vi "Download TBD file.vi"(8 "error in (no error)":errorcluster caption="错误输入（无错误）", 10 "TBC File Name":string="E100_TS2_23_90_V3.0.tbc", 11 "VISA资源名称":refnum<visa-resource-name>="COM1") -> (0 "错误输出":errorcluster, 2 "CMD In":string[](array[string]), 3 "Result":bool)   [LabVIEW 2013]
uses:
  C:/Program Files/National Instruments/LabVIEW 2013/examples/Instrument IO/Serial/support/Serial - Settings.ctl
  <vilib>/Instr/_visa.llb/VISA Configure Serial Port (Instr).vi
panel:
  out "读取缓冲区":string
  in  "文件路径（使用对话框）":path=path "E:/TBOX NEW/E100_TS2_23_90_V3.0.tbc"
  in  "TBC File Name 2":string="E100_TS2_23_90_V3.0.tbc"
  out "数组 2":bool[](array[boolean])
  out "添加的路径":path
  out "Feedback":string[](array[string])
  out "数组":string[](array[string])
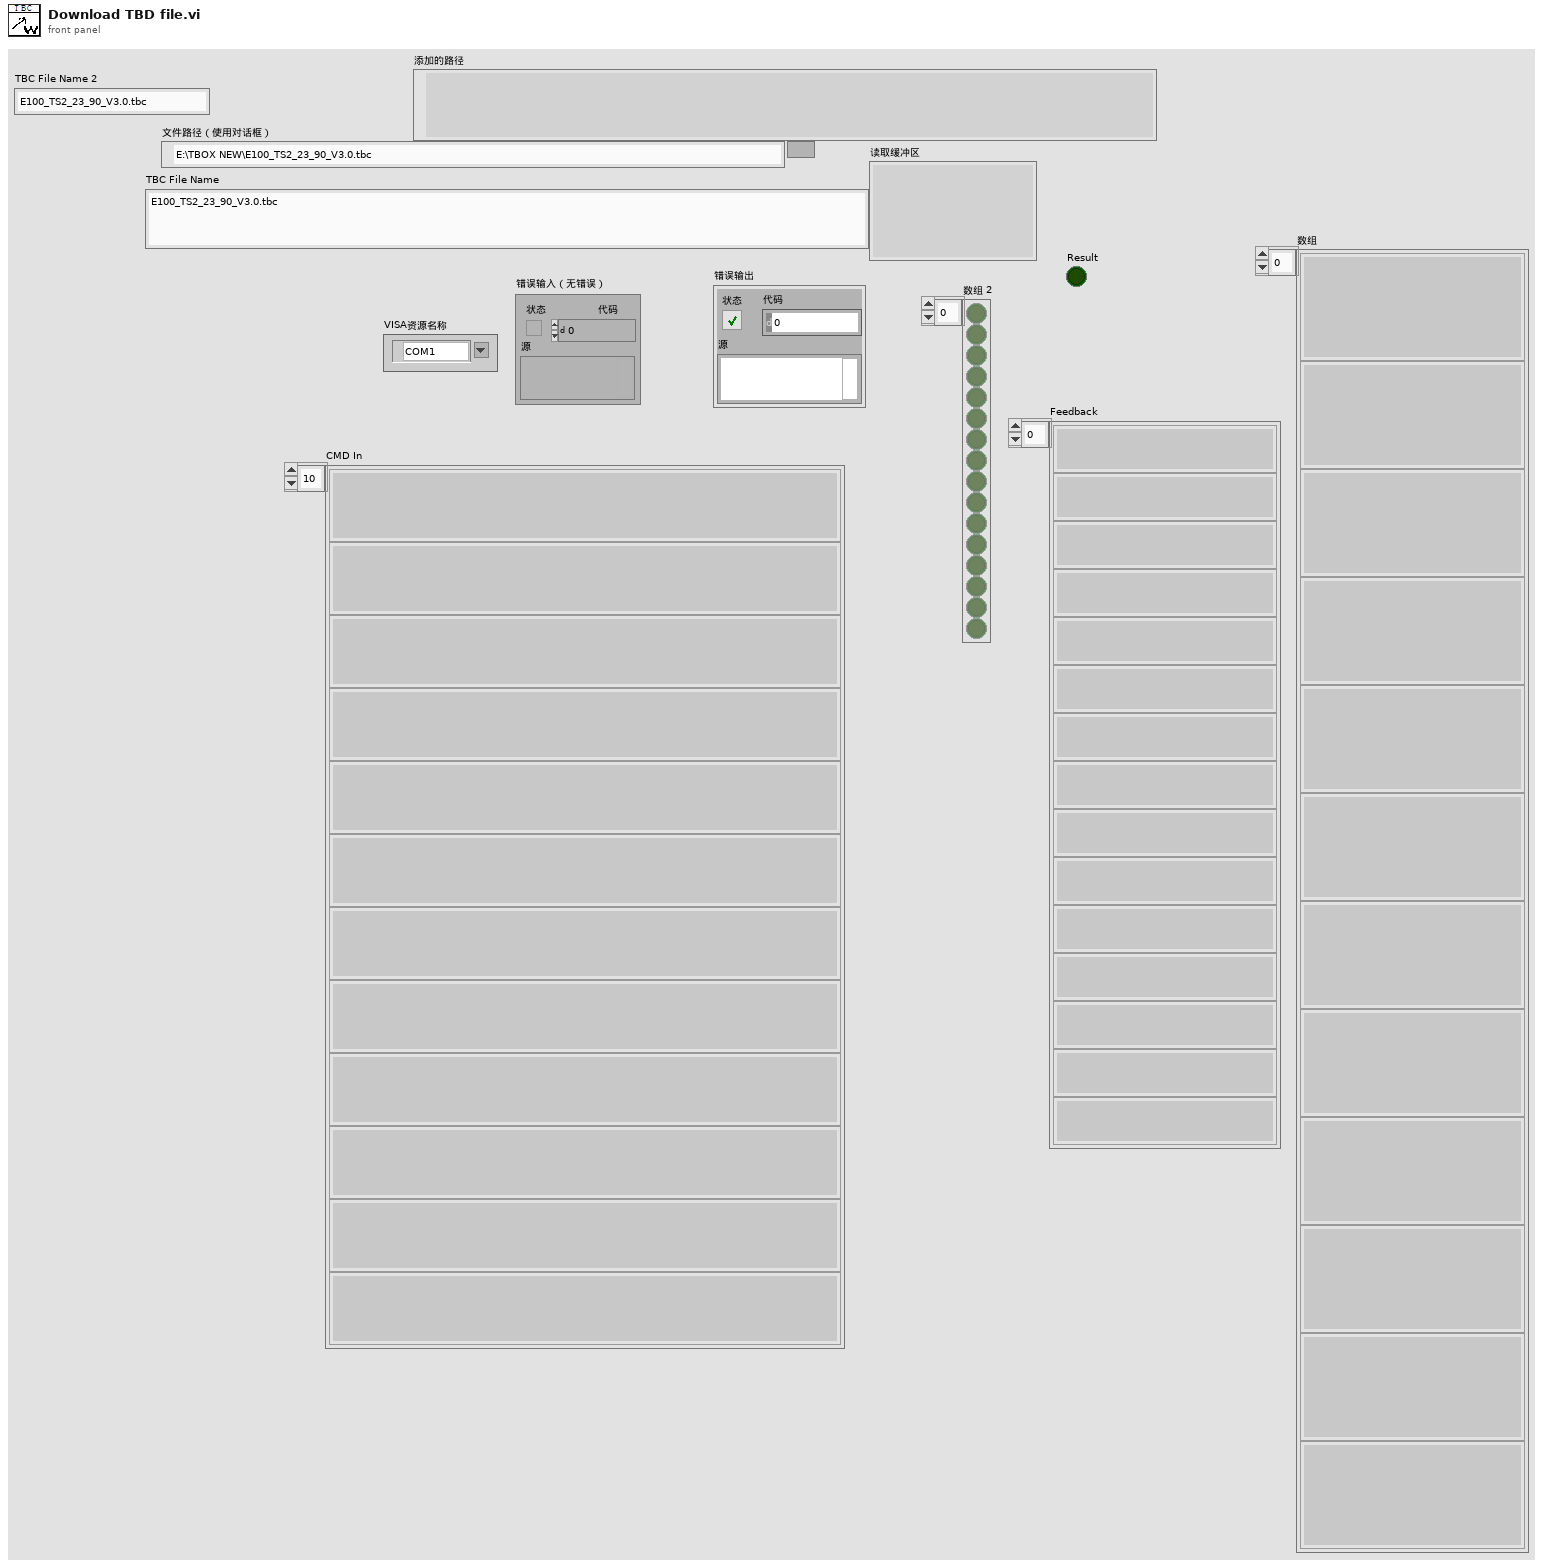
[diagram p1: front panel]
types:
  T1 = enum32{"invalid app kind", "Development System", "Run Time System", "Student Edition", "Embedded LabVIEW", "Evaluation", "Custom"}
  T2 = typedef "Serial - Settings.ctl" = cluster{"波特率":u32, "数据比特":u16, "奇偶":enum16{"None", "Odd", "Even", "Mark", "Space"}, "停止位":u16, "流控制":u16}
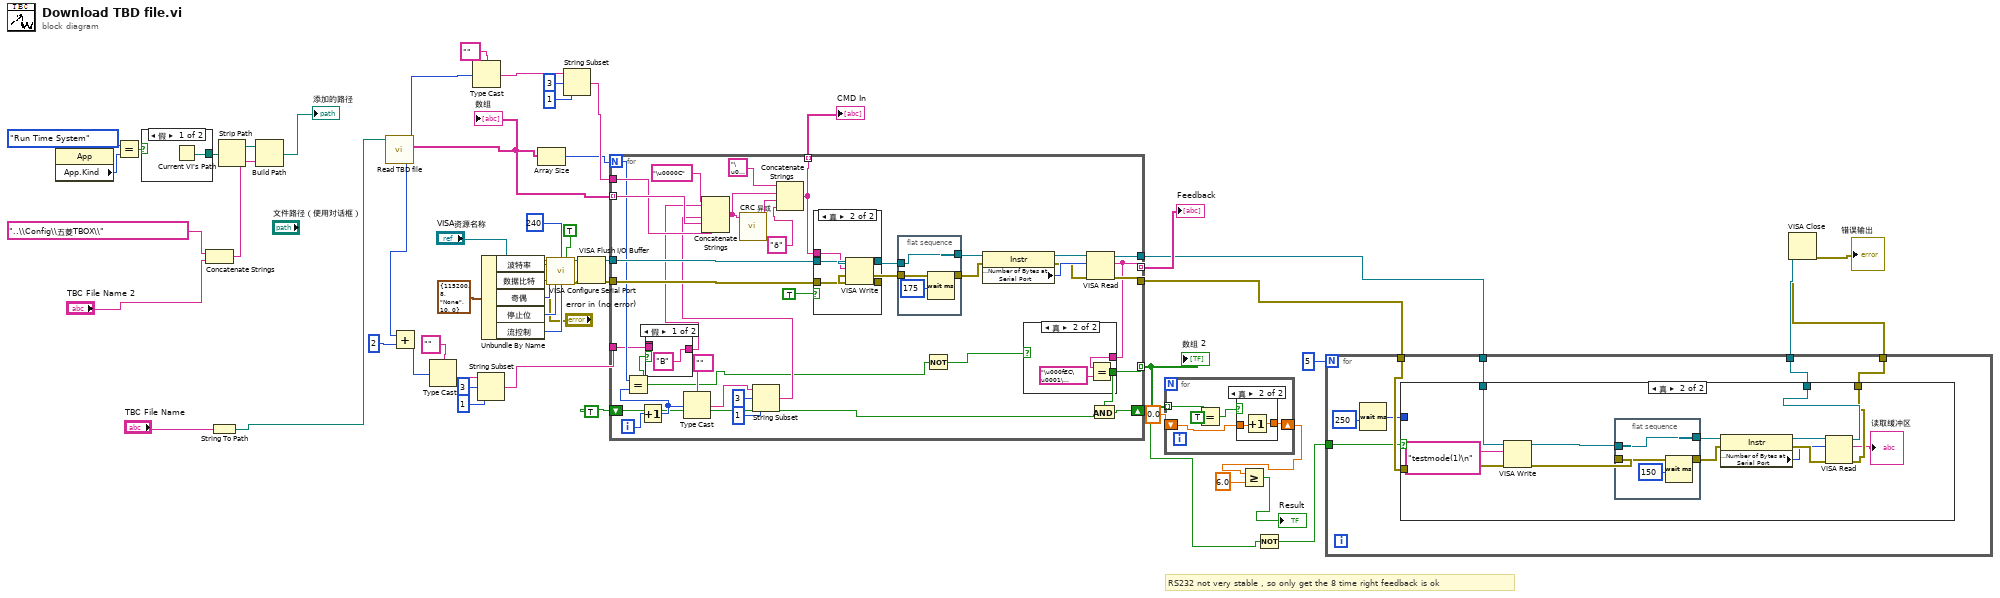
[diagram p0: block diagram]
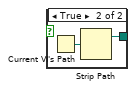
[diagram p4: hidden frame]
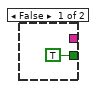
[diagram p5: hidden frame]
diagram:
  # "RS232 not very stable , so only get the 8 time right feedback is ok"
  n1 = property class="App"() -> ("App.Kind"=w23:T1)  [unwired: 2 in, 2 out]
  n2 = Equal?(x=T1."Run Time System" ("y"), y=w23) -> (x = y?=w25:bool)
  n3 = case shown="假" w25 {
    tunnel: [w58 w60] -> w24
    frame False {
      n4 = Current VI's Path() -> (path=w58:path)
    }
    frame True {
      n5 = Current VI's Path() -> (path=w59:path)
      n6 = Strip Path(path=w59) -> (stripped path=w60:path)  [unwired: 1 out]
    }
  }
  n7 = Concatenate Strings("..\\Config\\五菱TBOX\\" ("连接的字符串"), "TBC File Name 2") -> (w17:string)
  n8 = String To Path(string="TBC File Name") -> (path=w1:path)
  n9 = Strip Path(path=w24) -> (stripped path=w21:path)  [unwired: 1 out]
  n10 = Build Path(base path=w21, name or relative path=w17) -> (appended path=→"添加的路径":path)
  n11 = call "Read TBD file.vi"("文件路径（使用对话框）"=w1) -> ("末包数据量"=w27:i32, "数组"=w35:string[], "数据包数"=w41:i32)  [unwired: 7 in, 1 out]
  "数组" <- w35
  n12 = Add(x=w27, y=2 ("x-y*floor(x/y)")) -> (x+y=w28:i32)
  n13 = Type Cast(type="" ("类型"), x=w28) -> (*(type *) &x=w31:string)
  n14 = Type Cast(type="" ("类型"), x=w41) -> (*(type *) &x=w40:string)
  n15 = String Subset(string=w31, offset (0)=3 ("偏移量(0)"), length (rest)=1 ("长度（剩余）")) -> (substring=w29:string)
  n16 = Unbundle By Name(T2 {"波特率"=115200, "数据比特"=8, "奇偶"=enum."None", "停止位"=10, "流控制"=0} ("串口设置")) -> ("波特率"=w53:u32, "数据比特"=w54:u16, "奇偶"=w55:enum16{"None", "Odd", "Even", "Mark", "Space"}, "停止位"=w56:u16, "流控制"=w51:u16)
  n17 = Array Size(array=w35) -> (size(s)=w34:i32)
  n18 = call-poly "VISA Configure Serial Port"("VISA resource name"="VISA资源名称", "termination char\n(0xA = '\\n' = LF)"=u8 240 ("termination char\n(0xA = '\\n' = LF)"), "Enable Termination\nChar (T)"=TRUE ("Enable Termination\nChar (T)"), "baud rate (9600)"=w53, "data bits (8)"=w54, "parity (0:none)"=w55, "error in (no error)"="error in (no error)", "stop bits (10: 1 bit)"=w56, "flow control (0:none)"=w51) -> ("VISA resource name out"=w48:refnum<visa-resource-name>, "error out"=w49:errorcluster)  [unwired: 1 in, 4 out]
  n19 = String Subset(string=w40, offset (0)=3 ("偏移量(0)"), length (rest)=1 ("长度（剩余）")) -> (substring=w39:string)
  n20 = VISA Flush I/O Buffer(VISA resource name=w48, error in (no error)=w49) -> (VISA resource name out=w47:refnum<visa-resource-name>, error out=w46:errorcluster)  [unwired: 1 in]
  n21 = for {
    N: w34 -> [w75]
    tunnel: w47 -> [w96]
    tunnel: w46 -> [w95]
    tunnel: [w87] -> w11
    tunnel: [w86] -> w12
    tunnel: [w66] -> w44 mode=indexing
    tunnel: w35 -> [w84] mode=indexing
    tunnel: w39 -> [w81]
    tunnel: [w68] -> w36 mode=indexing
    tunnel: w29 -> [w74]
    shift-right: [w65] -> w2
    shift-left: TRUE -> [w64]
    tunnel: [w63] -> w8 mode=indexing
    i -> [w83]
    n22 = Increment(x=w83) -> (x+1=w76:i32)
    n23 = Equal?(x=w75, y=w76) -> (x = y?=w61:bool)
    n24 = case shown="假" w61 {
      tunnel: [_ w102] -> _
      tunnel: w74 -> [_ w102]
      tunnel: ["B" w102] -> w73
      frame False {
      }
      frame True {
      }
    }
    n25 = Type Cast(type="" ("类型"), x=w76) -> (*(type *) &x=w78:string)
    n26 = String Subset(string=w78, offset (0)=3 ("偏移量(0)"), length (rest)=1 ("长度（剩余）")) -> (substring=w77:string)
    n27 = Concatenate Strings("\u0000C", w73, w81, w77, w84) -> (w69:string)
    n28 = call "CRC 异或.vi"("input hex"=w69) -> ("*(类型 *) &x"=w71:string)  [unwired: 10 in]
    n29 = Concatenate Strings("\u000f" ("字符串"), w69, w71, "ð" ("字符串")) -> (w68:string)
    n30 = case shown="真" TRUE {
      tunnel: w96 -> [w107 w112]
      tunnel: [w107 w111] -> w94
      tunnel: [w106 w110] -> w92
      tunnel: w95 -> [w106 w109]
      tunnel: w68 -> [_ w108]
      frame False {
      }
      frame True {
        n31 = VISA Write(VISA resource name=w112, write buffer=w108, error in (no error)=w109) -> (VISA resource name out=w111:refnum<visa-resource-name>, error out=w110:errorcluster)  [unwired: 1 out]
      }
    }
    n32 = flat-sequence {
      tunnel: w92 -> [w105]
      tunnel: [w105] -> w91
      tunnel: w94 -> [w103]
      tunnel: [w103] -> w93
      frame #0 {
        n33 = Wait (ms)(milliseconds to wait=u32 175 ("等待时间（毫秒）")) -> ()  [unwired: 1 out]
      }
    }
    n34 = Not(x=w61) -> (.not. x?=w62:bool)
    n35 = property class="Instr"(reference=w93, error in=w91) -> (reference out=w88:refnum<visa-resource-name>, error out=w89:errorcluster, "Serial Settings:Number of Bytes at Serial Port"=w90:u32)
    n36 = VISA Read(VISA resource name=w88, byte count=w90, error in (no error)=w89) -> (VISA resource name out=w86:refnum<visa-resource-name>, read buffer=w66:string, error out=w87:errorcluster)  [unwired: 1 out]
    n37 = case shown="真" w62 {
      tunnel: w66 -> [_ w99]
      tunnel: [TRUE w98] -> w63
      frame False {
      }
      frame True {
        n38 = Equal?(x=w99, y="\u000f€C\u0001\u0001Âð") -> (x = y?=w98:bool)
      }
    }
    n39 = And(x=w63, y=w64) -> (x .and. y?=w65:bool)
  }
  "Feedback" <- w44
  "CMD In" <- w36
  "数组 2" <- w8
  n40 = for {
    tunnel: w8 -> [w116] mode=indexing
    shift-right: [w115] -> w6
    shift-left: 0.0 -> [w113]
    n41 = Equal?(x=w116, y=TRUE) -> (x = y?=w114:bool)
    n42 = case shown="真" w114 {
      tunnel: [w118 w120] -> w115
      tunnel: w113 -> [w118 w119]
      frame False {
      }
      frame True {
        n43 = Increment(x=w119) -> (x+1=w120:dbl)
      }
    }
  }
  n44 = Greater Or Equal?(x=w6, y=6.0) -> (x >= y?=→"Result":bool)
  n45 = Not(x=w2) -> (.not. x?=w3:bool)
  n46 = for {
    N: 5 -> [_]
    tunnel: w12 -> [w127]
    tunnel: w11 -> [w126]
    tunnel: [w125] -> w10
    tunnel: [w124] -> w9
    tunnel: w3 -> [w122]
    n47 = Wait (ms)(milliseconds to wait=u32 250 ("等待时间（毫秒）")) -> (millisecond timer value=w121:u32)
    n48 = case shown="真" w122 {
      tunnel: w127 -> [w129 w142]
      tunnel: w126 -> [w128 w140]
      tunnel: [w129 w132] -> w125
      tunnel: [w128 w131] -> w124
      tunnel: w121 -> [_ _]
      frame False {
      }
      frame True {
        n49 = VISA Write(VISA resource name=w142, write buffer="testmode(1)\n" ("写入缓冲区"), error in (no error)=w140) -> (VISA resource name out=w134:refnum<visa-resource-name>, error out=w133:errorcluster)  [unwired: 1 out]
        n50 = flat-sequence {
          tunnel: w133 -> [w145]
          tunnel: [w145] -> w136
          tunnel: w134 -> [w143]
          tunnel: [w143] -> w135
          frame #0 {
            n51 = Wait (ms)(milliseconds to wait=u32 150 ("等待时间（毫秒）")) -> ()  [unwired: 1 out]
          }
        }
        n52 = property class="Instr"(reference=w135, error in=w136) -> (reference out=w139:refnum<visa-resource-name>, error out=w138:errorcluster, "Serial Settings:Number of Bytes at Serial Port"=w137:u32)
        n53 = VISA Read(VISA resource name=w139, byte count=w137, error in (no error)=w138) -> (VISA resource name out=w132:refnum<visa-resource-name>, read buffer=→"读取缓冲区":string, error out=w131:errorcluster)  [unwired: 1 out]
      }
    }
  }
  n54 = VISA Close(VISA resource name=w10, error in (no error)=w9) -> (error out=→"错误输出":errorcluster)
